vi "GetAvailableTargets.vi"(8 "error in":errorcluster, 11 "Backend":T2) -> (0 "error out":errorcluster, 3 "Targets":T1[](array[typedef]))   [LabVIEW 2020, in "OpenLvVision_OpenCv.lvlib"]
doc: "Retruns for an backend the supported targets"
uses:
  OpenLvVision_OpenCv.lvlib
  TypeDef/Backend.ctl
  TypeDef/Target.ctl
  Dlls/OlvOpenCvWrapper.dll
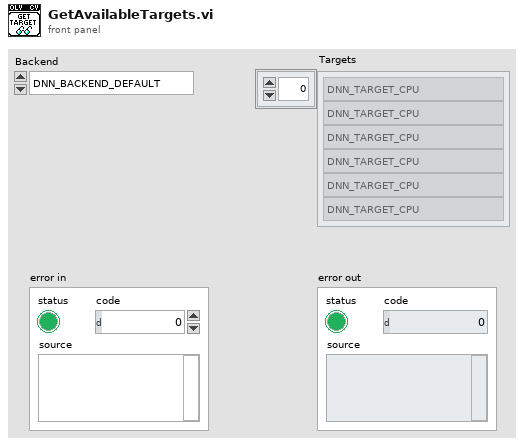
[diagram p1: front panel]
types:
  T1 = typedef "OpenLvVision_OpenCv.lvlib/Target.ctl" = enum16{"DNN_TARGET_CPU", "DNN_TARGET_OPENCL", "DNN_TARGET_OPENCL_FP16", "DNN_TARGET_MYRIAD", "DNN_TARGET_VULKAN", "DNN_TARGET_FPGA", "DNN_TARGET_CUDA", "DNN_TARGET_CUDA_FP16", "DNN_TARGET_HDDL", "DNN_TARGET_NPU", "DNN_TARGET_CPU_FP16"}
  T2 = typedef "OpenLvVision_OpenCv.lvlib/Backend.ctl" = enum16{"DNN_BACKEND_DEFAULT", "DNN_BACKEND_HALIDE", "DNN_BACKEND_INFERENCE_ENGINE", "DNN_BACKEND_OPENCV", "DNN_BACKEND_VKCOM", "DNN_BACKEND_CUDA", "DNN_BACKEND_WEBNN", "DNN_BACKEND_TIMVX", "DNN_BACKEND_CANN"}
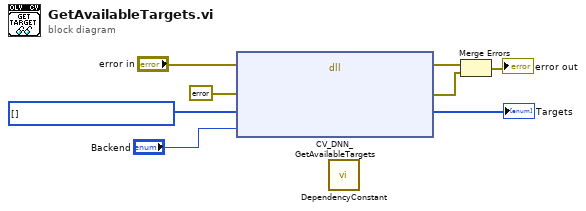
[diagram p0: block diagram]
diagram:
  w2 = T1[] [] items=["DNN_TARGET_CPU", "DNN_TARGET_OPENCL", "DNN_TARGET_OPENCL_FP16", "DNN_TARGET_MYRIAD", "DNN_TARGET_VULKAN", "DNN_TARGET_FPGA", "DNN_TARGET_CUDA", "DNN_TARGET_CUDA_FP16", "DNN_TARGET_HDDL", "DNN_TARGET_NPU", "DNN_TARGET_CPU_FP16"] ("Targets")
  n1 = dll-call lib="C:/Users/lukas/Downloads/OpenLvVision_OpenCv/SourceCode/LabView/OpenLvVision_OpenCv/Dlls/OlvOpenCvWrapper.dll" fn="CV_DNN_GetAvailableTargets"(error in="error in", "Error"=errorcluster {"status"=FALSE, "code"=0, "source"=""} ("error out"), "targetArrayHandle"=w2, "backend"="Backend") -> (error out=w7:errorcluster, "Error"=w5:errorcluster, "targetArrayHandle"=→"Targets":T1[])  [unwired: 4 in, 1 out]
  n2 = call "DependencyConstant.vi"() -> ()  [unwired: 12 in]
  n3 = Merge Errors(w7, w5) -> (→"error out":errorcluster)
